vi "from string.vi"(8 "error in":errorcluster, 9 "data":string, 10 "version":string, 11 "fixed channel configuration in":refnum<class "BuckBoost configuration.lvclass">) -> (0 "error out":errorcluster, 3 "fixed channel configuration out":refnum<class "BuckBoost configuration.lvclass">)   [LabVIEW 2017, in "BuckBoost configuration.lvclass"]
doc: "Provides an interface for loading a module configuration from a file or other serialized data source. It is recommended that all children of this class store data in two sets--data required for its own initialization, and any data required for parent initialization--and that each implementation uses the <b>Call Parent Method</b> primitive to de-serialize parent information. As a result, it is expected that every module configuration class calls <b>component configuration.lvclass:From String.vi</b>.\nNI Tag Bus Module Framework 1.0.3.43\nNI Systems Engineering"
uses:
  BuckBoost configuration.lvclass
  BuckBoost configuration.lvclass/BuckBoost configuration.ctl
  <vilib>/NI/JSON Support for LabVIEW/JSON Data Classes/JSON Helper/Parsing/Parse Value.vi
  <vilib>/NI/JSON Support for LabVIEW/JSON Data Classes/JSON Helper/To More Specific Type (Object).vi
  <vilib>/NI/JSON Support for LabVIEW/JSON Data Classes/JSON Object/Get Value (JSON).vi
  <vilib>/NI/JSON Support for LabVIEW/JSON Data Classes/JSON Datatype/JSON Null.lvclass
  <vilib>/NI/DCAF/Tag Editor Core/control module/configuration/control module configuration.lvclass
  <vilib>/NI/Configuration Framework/serializable configuration/NISE_CEF_serializable configuration.lvclass
  <vilib>/NI/JSON Support for LabVIEW/JSON Data Classes/JSON Helper/JSON Helper.lvclass
  <vilib>/NI/JSON Support for LabVIEW/JSON Data Classes/JSON Object/JSON Object.lvclass
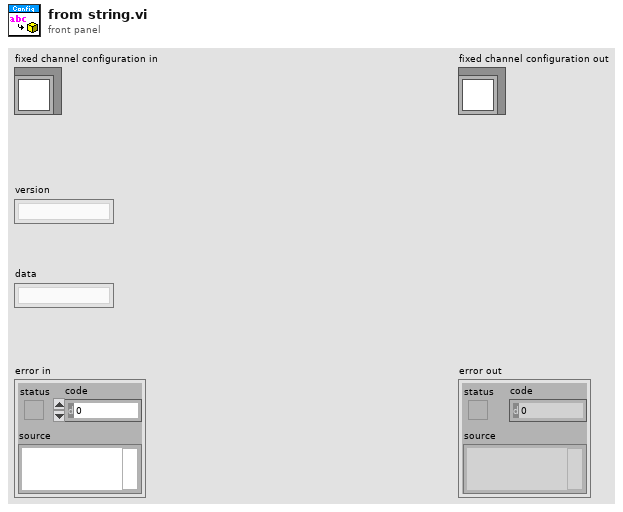
[diagram p1: front panel]
types:
  T1 = typedef "niFpgaPID_PIGains.ctl" = cluster{"proportional gain":sgl, "integral gain":sgl}
  T2 = typedef "BuckBoostInterface.lvlib/modulationConfig.ctl" = cluster{"SwitchingSpeed":dbl, "Deadband":dbl, "modulationRate":dbl}
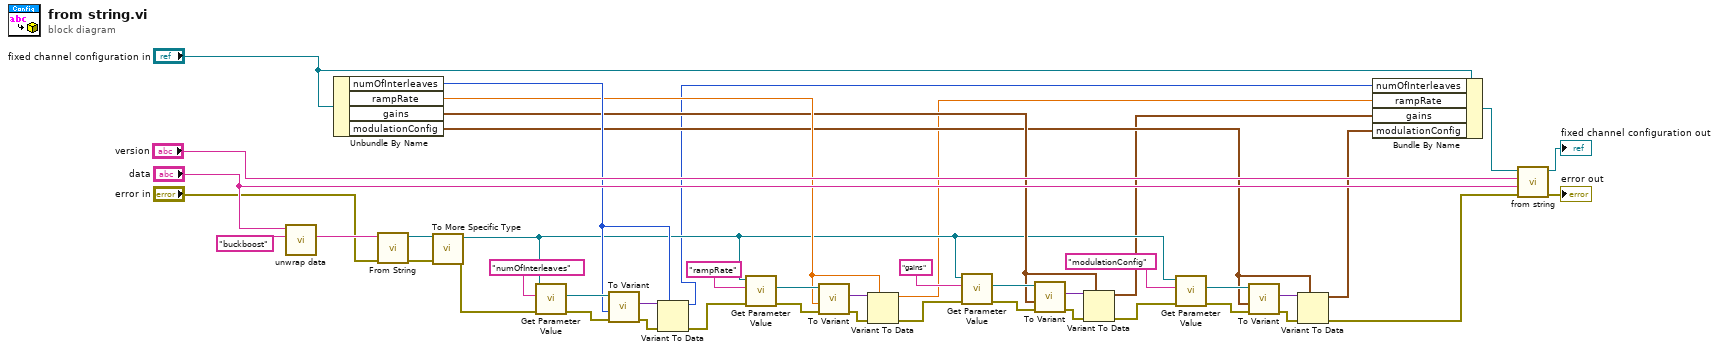
[diagram p0: block diagram]
diagram:
  n1 = call <vilib>:"unwrap data.vi"("identifier"="buckboost", "data to unwrap"="data") -> ("unwrapped data"=w41:string)  [unwired: 8 in, 1 out]
  n2 = Unbundle By Name("fixed channel configuration in") -> ("numOfInterleaves"=w30:u8, "rampRate"=w24:sgl, "gains"=w16:T1, "modulationConfig"=w8:T2)
  n3 = call <vilib>:"From String.vi"("error in (no error)"="error in", "JSON String"=w41) -> ("error out"=w37:errorcluster, "JSON out"=w40:refnum<class "JSON Null.lvclass">)  [unwired: 8 in]
  n4 = call-poly <vilib>:"To More Specific Type.vi"("error in (no error)"=w37, "JSON Datatype in"=w40) -> ("error out"=w36:errorcluster, "JSON Datatype out"=w9:refnum<class "JSON Object.lvclass">)  [unwired: 8 in]
  n5 = call-poly <vilib>:"Get Parameter Value.vi"("error in (no error)"=w36, "key"="numOfInterleaves", "JSON Object in"=w9) -> ("error out"=w33:errorcluster, "value"=w34:refnum<class "JSON Null.lvclass">)  [unwired: 7 in]
  n6 = call <vilib>:"To Variant.vi"("error in (no error)"=w33, "datatype and defaults"=w30, "JSON Datatype in"=w34) -> ("error out"=w31:errorcluster, "Variant"=w32:variant)  [unwired: 6 in, 1 out]
  n7 = Variant To Data(error in=w31, type=w30, Variant=w32) -> (data=w1:u8, error out=w25:errorcluster)
  n8 = call-poly <vilib>:"Get Parameter Value.vi"("error in (no error)"=w25, "key"="rampRate", "JSON Object in"=w9) -> ("error out"=w27:errorcluster, "value"=w26:refnum<class "JSON Null.lvclass">)  [unwired: 7 in]
  n9 = call <vilib>:"To Variant.vi"("error in (no error)"=w27, "datatype and defaults"=w24, "JSON Datatype in"=w26) -> ("error out"=w29:errorcluster, "Variant"=w28:variant)  [unwired: 6 in, 1 out]
  n10 = Variant To Data(error in=w29, type=w24, Variant=w28) -> (data=w2:sgl, error out=w18:errorcluster)
  n11 = call-poly <vilib>:"Get Parameter Value.vi"("error in (no error)"=w18, "key"="gains", "JSON Object in"=w9) -> ("error out"=w21:errorcluster, "value"=w22:refnum<class "JSON Null.lvclass">)  [unwired: 7 in]
  n12 = call <vilib>:"To Variant.vi"("error in (no error)"=w21, "datatype and defaults"=w16, "JSON Datatype in"=w22) -> ("error out"=w19:errorcluster, "Variant"=w20:variant)  [unwired: 6 in, 1 out]
  n13 = Variant To Data(error in=w19, type=w16, Variant=w20) -> (data=w3:T1, error out=w10:errorcluster)
  n14 = call-poly <vilib>:"Get Parameter Value.vi"("error in (no error)"=w10, "key"="modulationConfig", "JSON Object in"=w9) -> ("error out"=w12:errorcluster, "value"=w11:refnum<class "JSON Null.lvclass">)  [unwired: 7 in]
  n15 = call <vilib>:"To Variant.vi"("error in (no error)"=w12, "datatype and defaults"=w8, "JSON Datatype in"=w11) -> ("error out"=w14:errorcluster, "Variant"=w13:variant)  [unwired: 6 in, 1 out]
  n16 = Variant To Data(error in=w14, type=w8, Variant=w13) -> (data=w4:T2, error out=w7:errorcluster)
  n17 = Bundle By Name(cluster="fixed channel configuration in", "numOfInterleaves"=w1, "rampRate"=w2, "gains"=w3, "modulationConfig"=w4) -> (w5:refnum<class "BuckBoost configuration.lvclass">)
  n18 = call-parent <vilib>:"from string.vi"("error in"=w7, "data"="data", "version"="version", "fixed channel configuration in"=w5) -> ("error out"=→"error out":errorcluster, "fixed channel configuration out"=→"fixed channel configuration out":refnum<class "BuckBoost configuration.lvclass">)  [unwired: 6 in]
